vi "ComboBox - Convert Enum To String.vi"(1 "Display Order (enum)":T1) -> (0 "Display Order (ComboBox string)":string)   [LabVIEW 2023, in "Error Manager.lvlib"]
doc: "Blank VI with error handling."
uses:
  Error Manager.lvlib
  Display Order (enum).ctl
panel:
  # "Input\nInputs to the VI"
  # "Development\nControls or indicators that are useful for development or testing, but which are not outputs of the VI."
  # "Output\nOutputs of the VI"
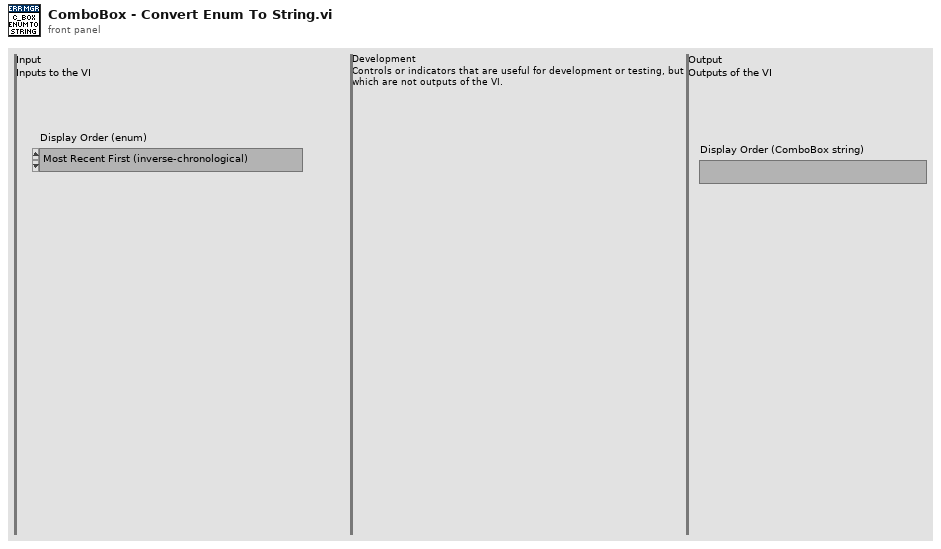
[diagram p1: front panel]
types:
  T1 = typedef "Error Manager.lvlib/Display Order (enum).ctl" = enum16{"Most Recent First (inverse-chronological)", "Oldest First (chronological)"}
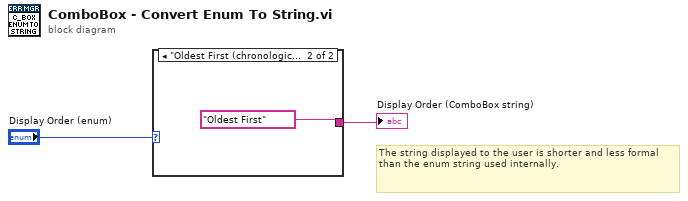
[diagram p0: block diagram]
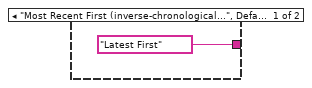
[diagram p2: hidden frame]
diagram:
  # "The string displayed to the user is shorter and less formal than the enum string used internally."
  n1 = case shown="\"Oldest First (chronological)\"" "Display Order (enum)" {
    tunnel: ["Latest First" "Oldest First"] -> w1
    frame "Most Recent First (inverse-chronological)", Default {
    }
    frame "Oldest First (chronological)" {
    }
  }
  "Display Order (ComboBox string)" <- w1
